vi "OMV_Close.vi"(8 "error in (no error)":errorcluster, 11 "Python":T1) -> ()   [LabVIEW 2022 SP3]
uses:
  PythonCtrl.ctl
  Processors.ctl
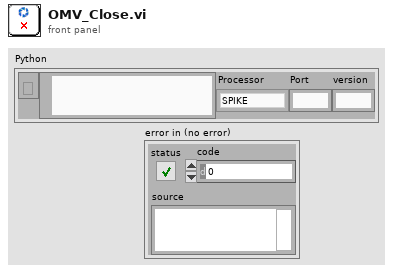
[diagram p1: front panel]
types:
  T1 = typedef "PythonCtrl.ctl" = cluster{"session":refnum<k35>, "PyPath":path, "Processor":T2, "Port":string, "version":string}
  T2 = typedef "Processors.ctl" = enum16{"SPIKE", "Pi", "Pi_ssh", "OpenMV", "Dunio"}
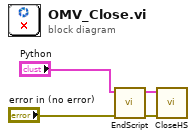
[diagram p0: block diagram]
diagram:
  n1 = call "EndScript.vi"("error in (no error)"="error in (no error)", "Python"="Python") -> ("error out"=w1:errorcluster, "Python"=w2:T1)  [unwired: 7 in, 1 out]
  n2 = call "CloseHS.vi"("error in (no error)"=w1, "Python"=w2) -> ()  [unwired: 10 in]
